vi "mag-field_stop_B-field.vi"(9 "mag fiel params":T1={"mag field"={"from"=16.0, "to"=5.0, "type"=enum."static"}, "use perm mode"=FALSE, "field info out"={"B field (consigne)"=16.648219020000003, "B field"=16.648219020000003, "B-field driver (vi reference)"=refnum, "consigne ctrl (driver)"=refnum, "field has arrived (ctrl, driver)"=refnum, "field  (ctrl, driver)"=refnum, "Coil supply"=refnum, "GPIB adress"=refnum}, "GPIB adr"="", "driver running?"=FALSE, "ON?"=FALSE, "Coil_Information"={"Max Field 10V Input"=0.0, "Waiting time for 0.5mT step"=0.0, "Dac_Output_Channel"=""}}) -> ()   [LabVIEW 2010]
uses:
  mag-field-control.ctl
  type defs - instruments/sweep info.ctl
  type defs - instruments/usage.ctl
  field-info.ctl
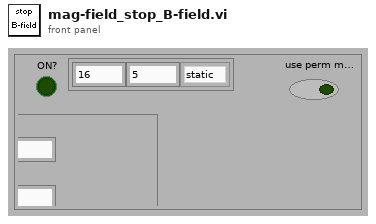
[diagram p1: front panel]
types:
  T1 = typedef "mag-field-control.ctl" = cluster{"mag field":T2, "use perm mode":bool, "field info out":T4, "GPIB adr":string, "driver running?":bool, "ON?":bool, "Coil_Information":cluster{"Max Field 10V Input":dbl, "Waiting time for 0.5mT step":dbl, "Dac_Output_Channel":tag}}
  T2 = typedef "sweep info.ctl" = cluster{"from":sgl, "to":sgl, "type":T3}
  T3 = typedef "usage.ctl" = enum8{"static", "sweep", "step", "step 2", "step 3"}
  T4 = typedef "field-info.ctl" = cluster{"B field (consigne)":dbl, "B field":dbl, "B-field driver (vi reference)":refnum<vi>, "consigne ctrl (driver)":refnum<vi>, "field has arrived (ctrl, driver)":refnum<vi>, "field  (ctrl, driver)":refnum<vi>, "Coil supply":refnum<vi>, "GPIB adress":refnum<vi>}
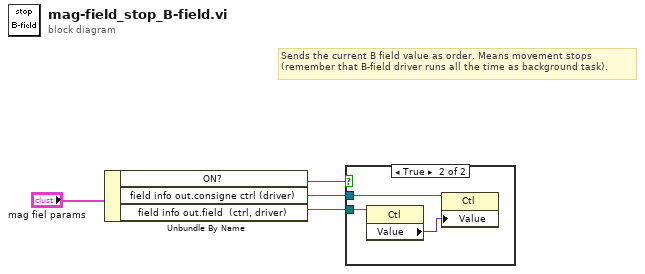
[diagram p0: block diagram]
diagram:
  # "Sends the current B field value as order. Means movement stops\n(remember that B-field driver runs all the time as background task)."
  n1 = Unbundle By Name("mag fiel params") -> ("ON?"=w1:bool, "field info out.consigne ctrl (driver)"=w2:refnum<vi>, "field info out.field  (ctrl, driver)"=w3:refnum<vi>)
  n2 = case shown="True" w1 {
    tunnel: w3 -> [_ w7]
    tunnel: w2 -> [_ w6]
    frame False {
    }
    frame True {
      n3 = property class="Ctl"(reference=w7) -> ("Value"=w5:variant)  [unwired: 1 in, 2 out]
      n4 = property class="Ctl"(reference=w6, "Value"=w5) -> ()  [unwired: 1 in, 2 out]
    }
  }
